vi "Draw Nav Pic.vi"(8 "Error In":errorcluster, 11 "Pane Relief Main UI in":refnum<class "Pane Relief Main UI.lvclass">) -> (0 "Error Out":errorcluster, 3 "Pane Relief Main UI out":refnum<class "Pane Relief Main UI.lvclass">)   [LabVIEW 2018, in "Pane Relief Main UI.lvlib" / "Pane Relief Main UI.lvclass"]
uses:
  <resource>/dialog/QuickDrop/plugins/PaneRelief/Classes/Pane Relief Main UI/Pane Relief Main UI/Pane Relief Main UI.lvclass
  <resource>/dialog/QuickDrop/plugins/PaneRelief/Classes/Pane Relief Main UI/Pane Relief Main UI/Pane Relief Main UI.lvclass/Pane Relief Main UI.ctl
  <resource>/dialog/QuickDrop/plugins/PaneRelief/Classes/Panel Object/Panel Object.lvclass
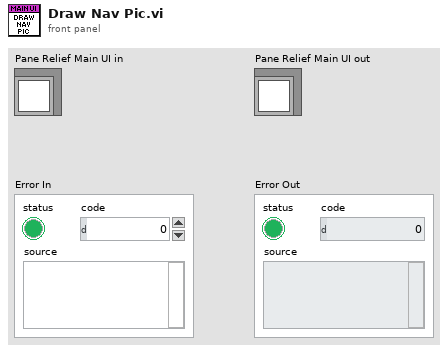
[diagram p1: front panel]
types:
  T1 = typedef "Point--Cluster.ctl" = cluster{"Horizontal":i32, "Vertical":i32}
  T2 = typedef "imagedata.ctl" = cluster{"image type":i32, "image depth":i32, "image":u8[], "mask":u8[], "colors":u32[], "Rectangle":cluster{"left":i16, "top":i16, "right":i16, "bottom":i16}}
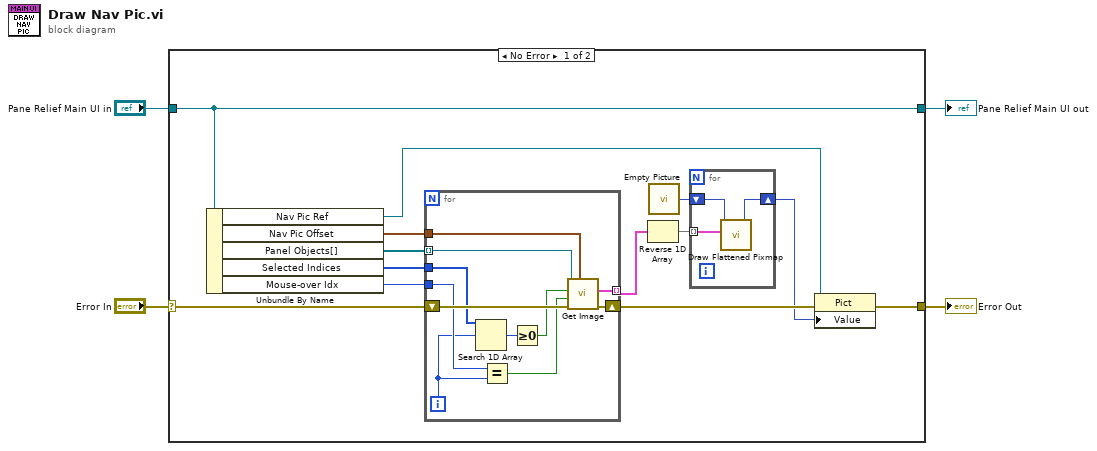
[diagram p0: block diagram]
diagram:
  n1 = case shown="No Error" "Error In" {
    selector: "Error In" -> [w9 w33]
    tunnel: [w7 w33] -> w1
    tunnel: [w10 w32] -> w3
    tunnel: "Pane Relief Main UI in" -> [w10 w32]
    frame No Error {
      n2 = Unbundle By Name(w10) -> ("Nav Pic Ref"=w6:refnum<vi>, "Nav Pic Offset"=w16:T1, "Panel Objects[]"=w17:refnum<class "Panel Object.lvclass">[], "Selected Indices"=w13:i32[], "Mouse-over Idx"=w12:i32)
      n3 = for {
        tunnel: w17 -> [w25] mode=indexing
        shift-right: [w30] -> w8
        shift-left: w9 -> [w31]
        tunnel: w16 -> [w26]
        tunnel: [w29] -> w15 mode=indexing
        tunnel: w13 -> [w24]
        tunnel: w12 -> [w28]
        i -> [w23]
        n4 = Search 1D Array(1D array=w24, element=w23) -> (index of element=w22:i32)  [unwired: 1 in]
        n5 = Equal?(x=w28, y=w23) -> (x = y?=w27:bool)
        n6 = Greater Or Equal To 0?(x=w22) -> (x >= 0?=w21:bool)
        n7 = call-dynamic "Get Image.vi"("Offset"=w26, "Error In"=w31, "Mouse-over"=w27, "Selected"=w21, "Panel Object in"=w25) -> ("Error Out"=w30:errorcluster, "Image"=w29:T2)  [unwired: 4 in, 1 out]
      }
      n8 = Reverse 1D Array(array=w15) -> (reversed array=w14:T2[])
      n9 = call "Empty Picture"() -> ("empty picture"=w11:picture)
      n10 = for {
        tunnel: w14 -> [w20] mode=indexing
        shift-right: [w18] -> w5
        shift-left: w11 -> [w19]
        n11 = call <vilib>:"Draw Flattened Pixmap.vi"("image data"=w20, "picture"=w19) -> ("new picture"=w18:picture)  [unwired: 7 in]
      }
      n12 = property class="Pict"(reference=w6, error in=w8, "Value"=w5) -> (error out=w7:errorcluster)  [unwired: 1 out]
    }
    frame Error {
    }
  }
  "Pane Relief Main UI out" <- w3
  "Error Out" <- w1
